vi "Waveform Resample.vi"() -> ()   [LabVIEW 2013]
panel:
  in  "stop":bool
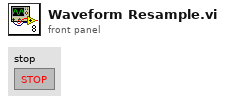
[diagram p1: front panel]
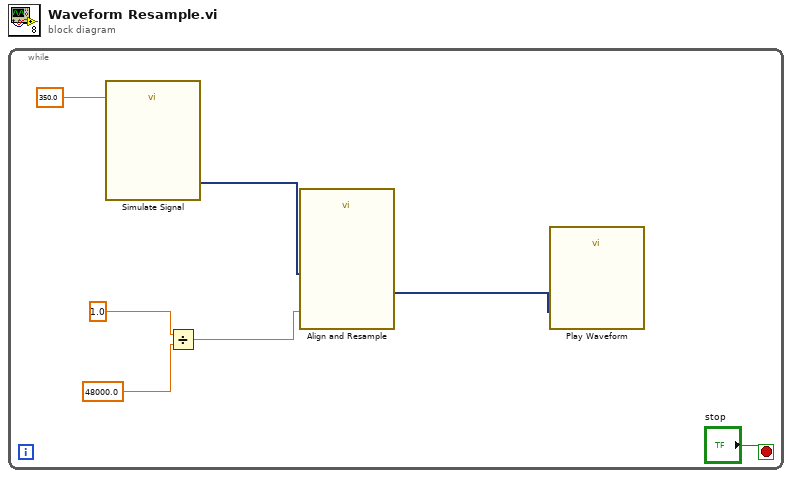
[diagram p0: block diagram]
diagram:
  n1 = while {
    stop <- "stop" stop-if-true
    n2 = call "Simulate Signal"("Frequency"=350.0) -> ("Sine"=w3:dynamicdata)  [unwired: 13 in, 1 out]
    n3 = Divide(x=1.0, y=48000.0) -> (x/y=w2:dbl)
    n4 = call "Align and Resample"("dt"=w2, "Signals"=w3) -> ("Resampled Signals"=w1:dynamicdata)  [unwired: 7 in, 2 out]
    n5 = call "Play Waveform"("Data"=w1) -> ()  [unwired: 18 in, 1 out]
  }
